vi "CreateSNRegistryKey.vi"() -> ()   [LabVIEW 2017]
uses:
  <vilib>/registry/registry.llb/Registry RtKey.ctl
  <vilib>/registry/registry.llb/Write Registry Value Simple.vi
panel:
  out "error out 2":errorcluster
  out "error out":errorcluster
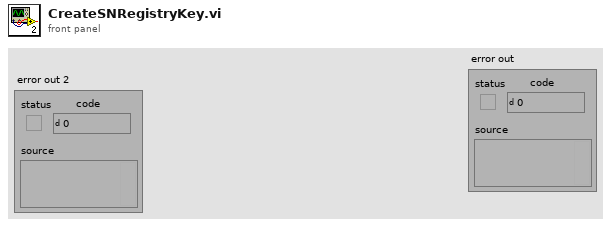
[diagram p1: front panel]
types:
  T1 = typedef "Registry RtKey.ctl" = enum32{"HKEY_CLASSES_ROOT", "HKEY_CURRENT_USER", "HKEY_LOCAL_MACHINE", "HKEY_USERS", "HKEY_PERFORMANCE_DATA", "HKEY_CURRENT_CONFIG", "HKEY_DYN_DATA"}
  T2 = typedef "Registry refnum.ctl" = refnum<k1>
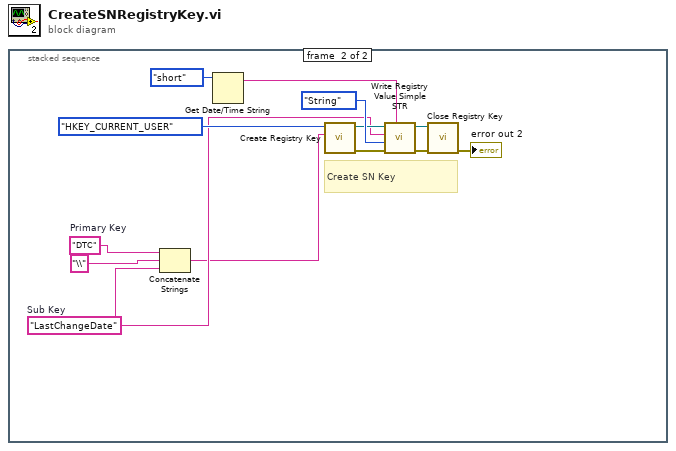
[diagram p0: block diagram]
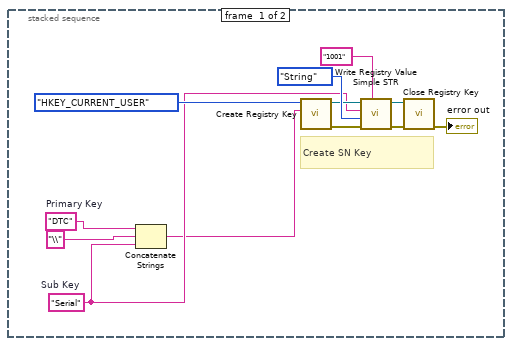
[diagram p2: hidden frame]
diagram:
  n1 = stacked-sequence {
    frame #0 {
      w5 = "DTC"  # Primary Key
      w3 = "Serial"  # Sub Key
      # "Create SN Key"
      n2 = Concatenate Strings(w5, "\\", w3) -> (w2:string)
      n3 = call <vilib>:"Create Registry Key.vi"("subkey"=w2, "root key (HKEY_LOCAL_MACHINE)"=Registry_RtKey."HKEY_CURRENT_USER") -> ("error out"=w10:errorcluster, "refnum out"=w8:T2)  [unwired: 7 in, 1 out]
      n4 = call-poly <vilib>:"Write Registry Value Simple STR.vi"("String/Binary data"="1001", "error in (no error)"=w10, "simple data type"=enum16{"String", "Binary", "DWORD"}."String", "value"=w3, "refnum"=w8) -> ("error out"=w12:errorcluster, "refnum out"=w11:T2)  [unwired: 3 in]
      n5 = call <vilib>:"Close Registry Key.vi"("error in (no error)"=w12, "refnum"=w11) -> ("error out"=→"error out":errorcluster)  [unwired: 5 in]
    }
    frame #1 {
      w19 = "DTC"  # Primary Key
      w17 = "LastChangeDate"  # Sub Key
      # "Create SN Key"
      n6 = Concatenate Strings(w19, "\\", w17) -> (w16:string)
      n7 = Get Date/Time String(date format (0)=enum16{"short", "long", "abbreviated"}."short") -> (date string=w13:string)  [unwired: 2 in, 1 out]
      n8 = call <vilib>:"Create Registry Key.vi"("subkey"=w16, "root key (HKEY_LOCAL_MACHINE)"=Registry_RtKey."HKEY_CURRENT_USER") -> ("error out"=w23:errorcluster, "refnum out"=w21:T2)  [unwired: 7 in, 1 out]
      n9 = call-poly <vilib>:"Write Registry Value Simple STR.vi"("String/Binary data"=w13, "error in (no error)"=w23, "simple data type"=enum16{"String", "Binary", "DWORD"}."String", "value"=w17, "refnum"=w21) -> ("error out"=w25:errorcluster, "refnum out"=w24:T2)  [unwired: 3 in]
      n10 = call <vilib>:"Close Registry Key.vi"("error in (no error)"=w25, "refnum"=w24) -> ("error out"=→"error out 2":errorcluster)  [unwired: 5 in]
    }
  }
